vi "Configure Data Format.vi"(8 "error in (no error)":errorcluster, 9 "Set Byte Order (0: Normal)":i32(ring) items=["Normal", "Swapped"], 10 "Data Format (0: ASCII)":i32(ring) items=["ASCII", "REAL"], 11 "VISA resource name":refnum<visa-resource-name>) -> (0 "error out":errorcluster, 3 "VISA resource name out":refnum<visa-resource-name>)   [LabVIEW 2011, in "Agilent N432A.lvlib"]
doc: "Sets the data format for transferring numeric information."
uses:
  <instrlib>/Agilent N432A/Agilent N432A.lvlib
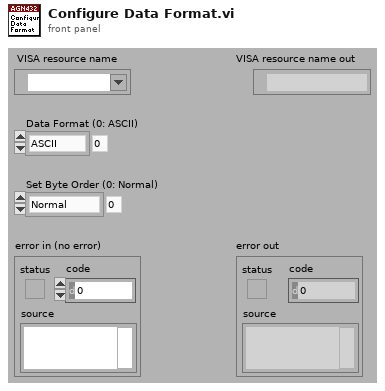
[diagram p1: front panel]
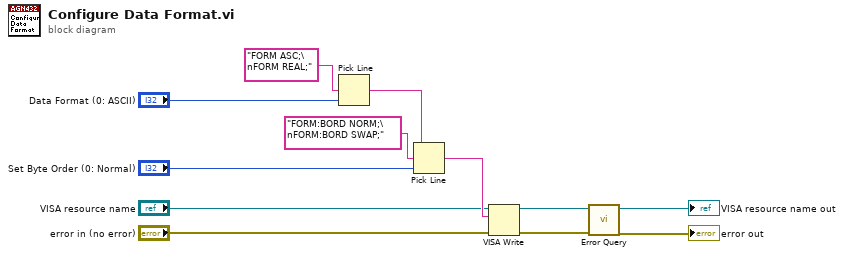
[diagram p0: block diagram]
diagram:
  n1 = Pick Line(multi-line string="FORM ASC;\nFORM REAL;", line index="Data Format (0: ASCII)") -> (output string=w8:string)  [unwired: 1 in]
  n2 = Pick Line(string ("")=w8, multi-line string="FORM:BORD NORM;\nFORM:BORD SWAP;", line index="Set Byte Order (0: Normal)") -> (output string=w7:string)
  n3 = VISA Write(VISA resource name="VISA resource name", write buffer=w7, error in (no error)="error in (no error)") -> (VISA resource name out=w4:refnum<visa-resource-name>, error out=w3:errorcluster)  [unwired: 1 out]
  n4 = call <instrlib>:"Error Query.vi"("error in (no error)"=w3, "VISA resource name"=w4) -> ("error out"=→"error out":errorcluster, "VISA resource name out"=→"VISA resource name out":refnum<visa-resource-name>)  [unwired: 6 in, 2 out]
